vi "Grid Pattern Dialog.vi"(8 "error in (no error)":errorcluster, 10 "Fixed Shape?":bool, 11 "Grid Settings In":T1={"Grid Type"=enum."Single Point", "Complex Convention"=enum."Re / Im", "Pattern Type"=enum."Rectangular", "Major Order Index"=0, "Grid Settings Value 1"=0.0+0.0i, "Grid Settings Value 2"=0.0+0.0i, "Pattern Settings Value 1"=0, "Pattern Settings Value 2"=0, "Values"=[0.0+0.0i]}) -> (0 "error out":errorcluster, 1 "Cancelled?":bool, 2 "Values":cdb[](array[numeric]), 3 "Grid Settings Out":T1={"Grid Type"=enum."Single Point", "Complex Convention"=enum."Re / Im", "Pattern Type"=enum."Rectangular", "Major Order Index"=0, "Grid Settings Value 1"=0.0+0.0i, "Grid Settings Value 2"=0.0+0.0i, "Pattern Settings Value 1"=0, "Pattern Settings Value 2"=0, "Values"=[0.0+0.0i]})   [LabVIEW 2023, in "NI_HFNetworkAnalysis.lvlib"]
doc: "Dialog box to define a grid pattern of complex values on a Smith Chart."
uses:
  NI_HFNetworkAnalysis.lvlib
  Controls/GridSettings.ctl
  Controls/ComplexConvention.ctl
  Controls/GridPatternType.ctl
  <vilib>/Utility/miscctls.llb/LVRowAndColumnTypeDef.ctl
  <vilib>/picture/smith.llb/Smith Plot Style.ctl
panel:
  in  "Right Panel":enum32{"Page 2"}(tab)
  out "Smith Chart":picture
  in  "Left Panel":enum32{"Page 1", "Page 3"}(tab)
  in  "Grid Settings":T4 caption="Grid"
  in  "Pattern Settings":cluster{"value1":u32, "value2":u32}={"value1"=1, "value2"=1} caption="Pattern" {"value2" min=1; "value1" min=1}
  in  "Point":T5
  out "Custom Grid":string[][](table)
  in  "Cancel Button":bool
  in  "OK Button":bool
  in  "Order":u16(ring) caption="Order:" items=["Amp slowest", "Pha slowest"]
  in  "Shape Type":u16(ring) caption="Shape:" items=["Single Point", "Rectangle", "Circle", "Pie", "Custom"]
  in  "Pattern Type":u16(ring) caption="Format:" items=["Re / Im", "Amp / Pha"]
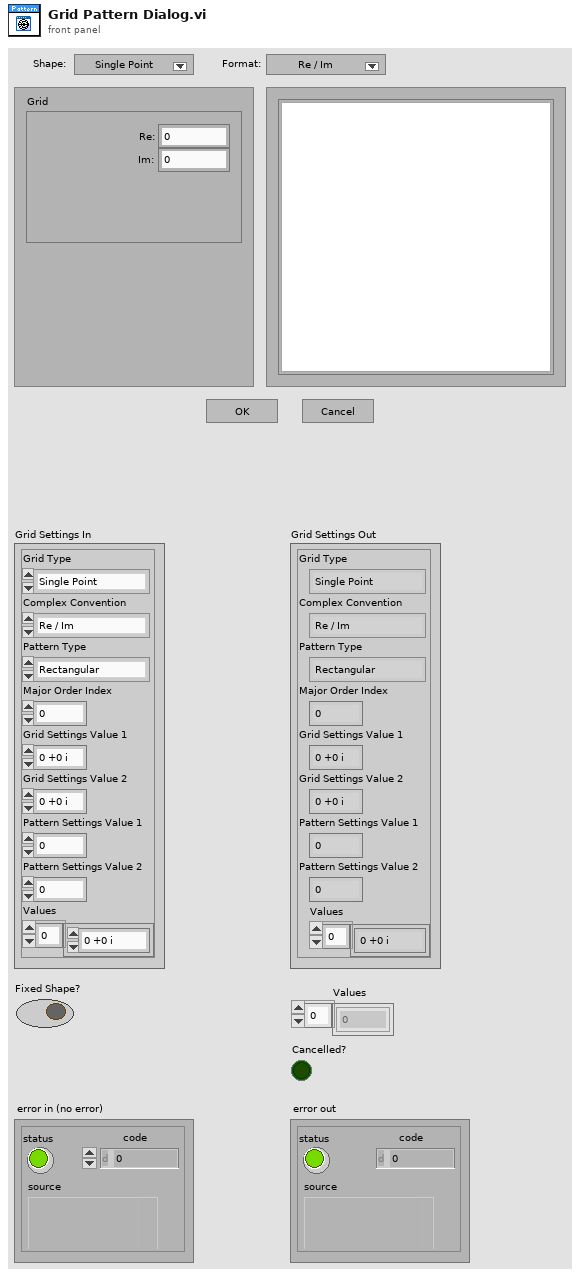
[diagram p1: front panel]
types:
  T1 = typedef "NI_HFNetworkAnalysis.lvlib/GridSettings.ctl" = cluster{"Grid Type":enum16{"Single Point", "Rectangle", "Circle", "Pie", "Custom"}, "Complex Convention":T2, "Pattern Type":T3, "Major Order Index":i32, "Grid Settings Value 1":cdb, "Grid Settings Value 2":cdb, "Pattern Settings Value 1":u32, "Pattern Settings Value 2":u32, "Values":cdb[]}
  T2 = typedef "NI_HFNetworkAnalysis.lvlib/ComplexConvention.ctl" = enum16{"Re / Im", "Amp / Pha"}
  T3 = typedef "NI_HFNetworkAnalysis.lvlib/GridPatternType.ctl" = enum16{"Rectangular", "Circular", "Undefined"}
  T4 = cluster{"value1":dbl, "value2":dbl, "value3":dbl, "value4":dbl}
  T5 = cluster{"value1":dbl, "value2":dbl, "Delete Point":bool, "Add Point":bool}
  T6 = enum16{"Single Point", "Rectangle", "Circle", "Pie", "Custom"}
  T7 = cluster{"# Horiz Points:":dbl, "# Vert Points:":dbl, "Delete Point":bool, "Add Point":bool}
  T8 = typedef "LVRowAndColumnTypeDef.ctl" = cluster{"Row":i32, "Column":i32}
  T9 = enum8{"Enabled", "Disabled", "Disabled and Grayed Out"}
  T10 = cluster{"x minimum":dbl, "x maximum":dbl, "y minimum":dbl, "y maximum":dbl}
  T11 = typedef "Smith Plot Style.ctl" = u16
  T12 = cluster{"Plot Style":T11, "Line Color":u32, "Point Color":u32}
  T13 = cluster{"R color":u32, "R grids":bool, "X color":u32, "X grids":bool, "Labels":bool}
  T14 = typedef "LVBoundsTypeDef.ctl" = cluster{"Width":u32, "Height":u32}
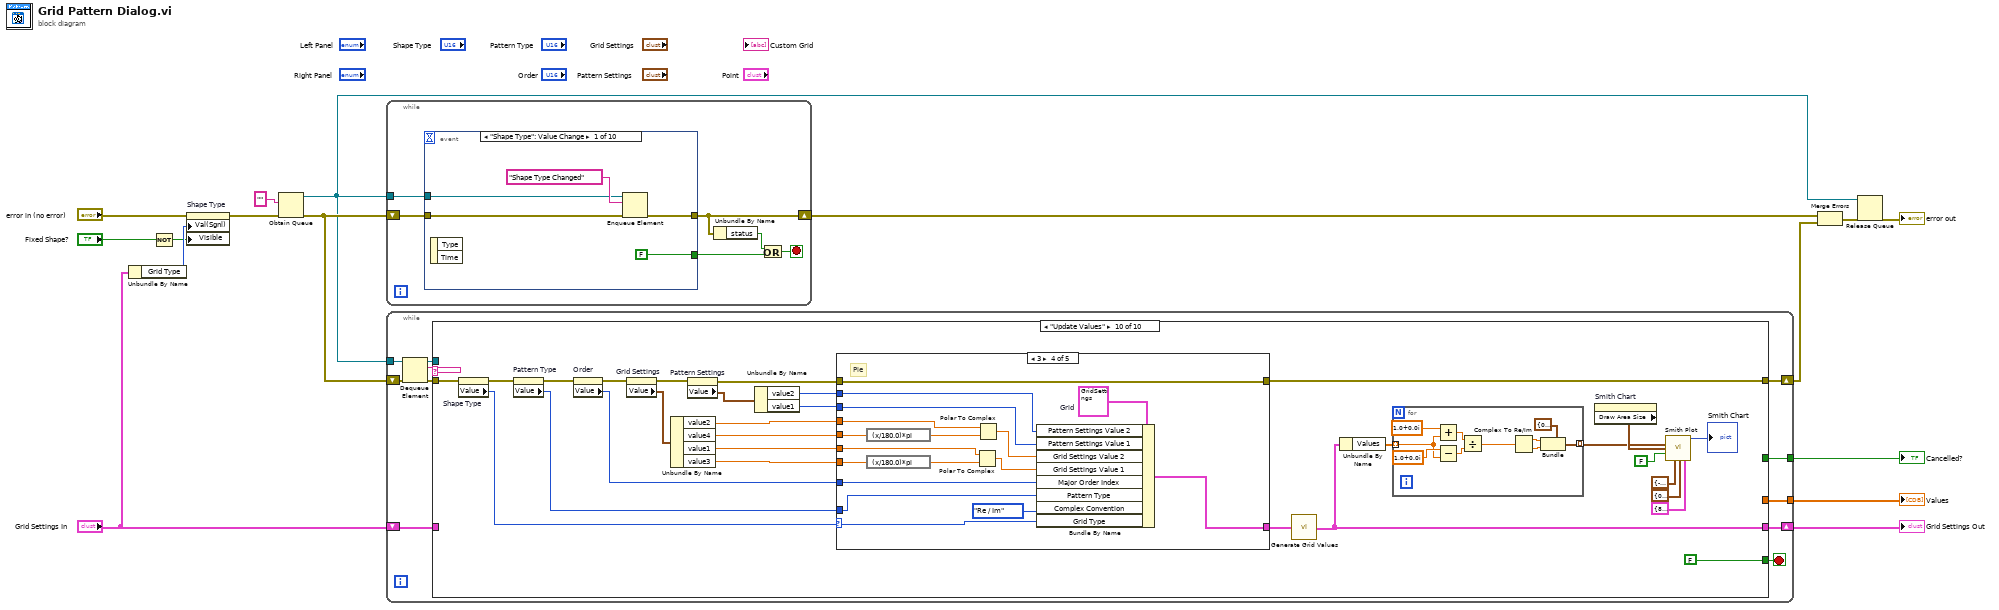
[diagram p0: block diagram]
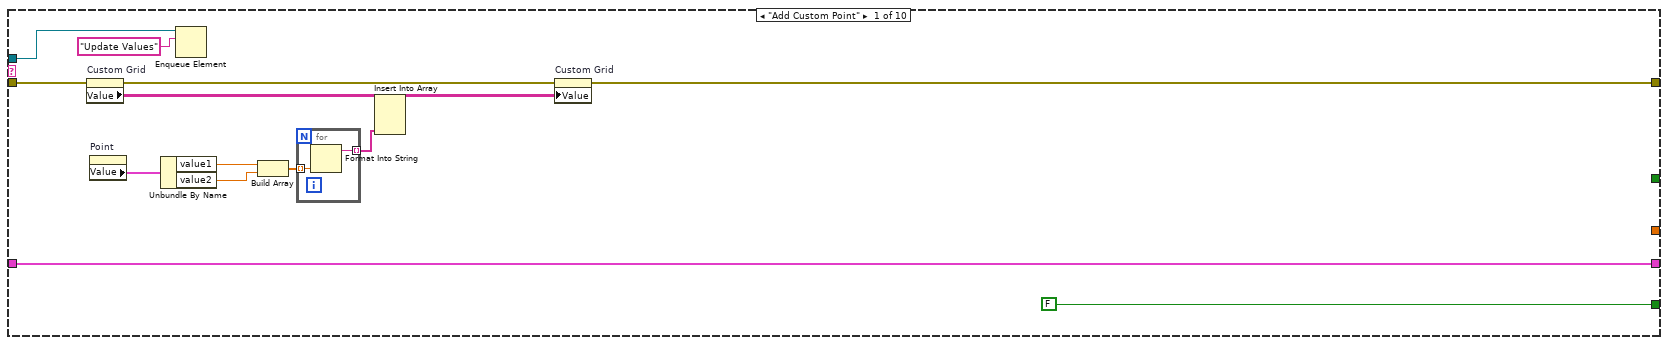
[diagram p2: hidden frame]
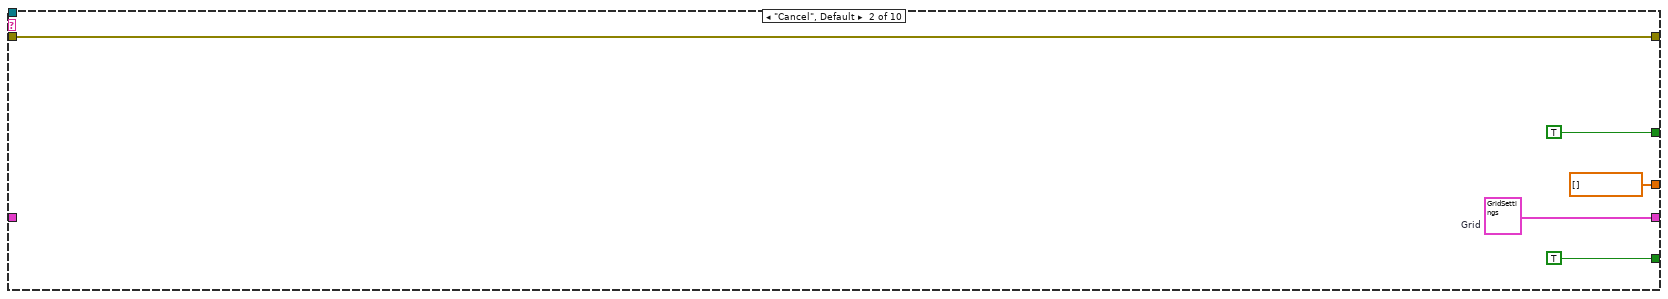
[diagram p3: hidden frame]
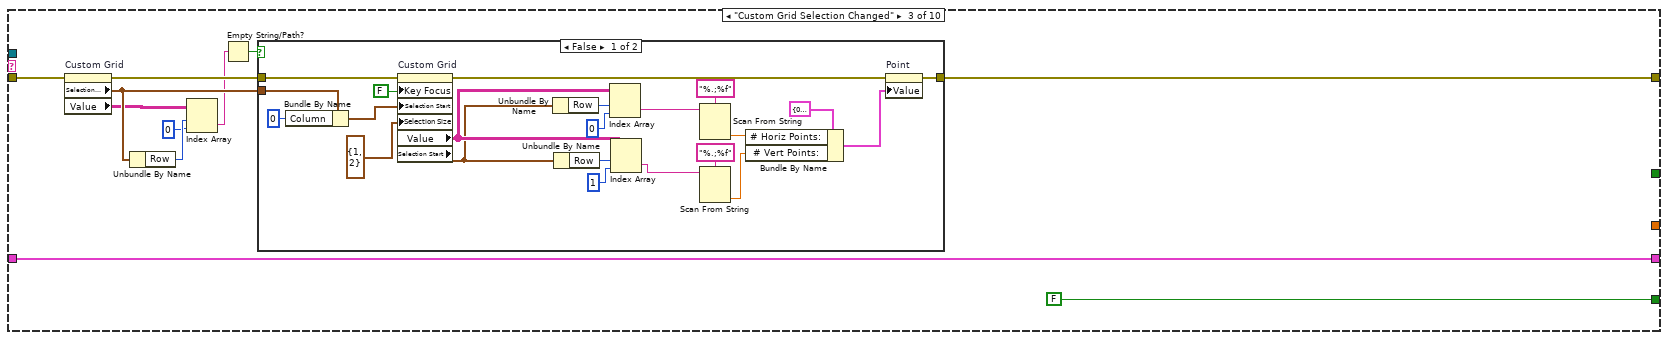
[diagram p4: hidden frame]
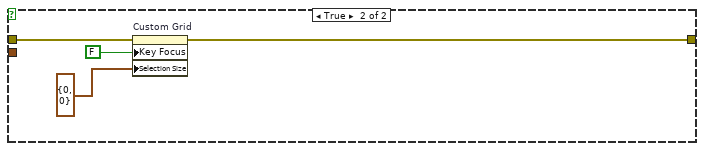
[diagram p5: hidden frame]
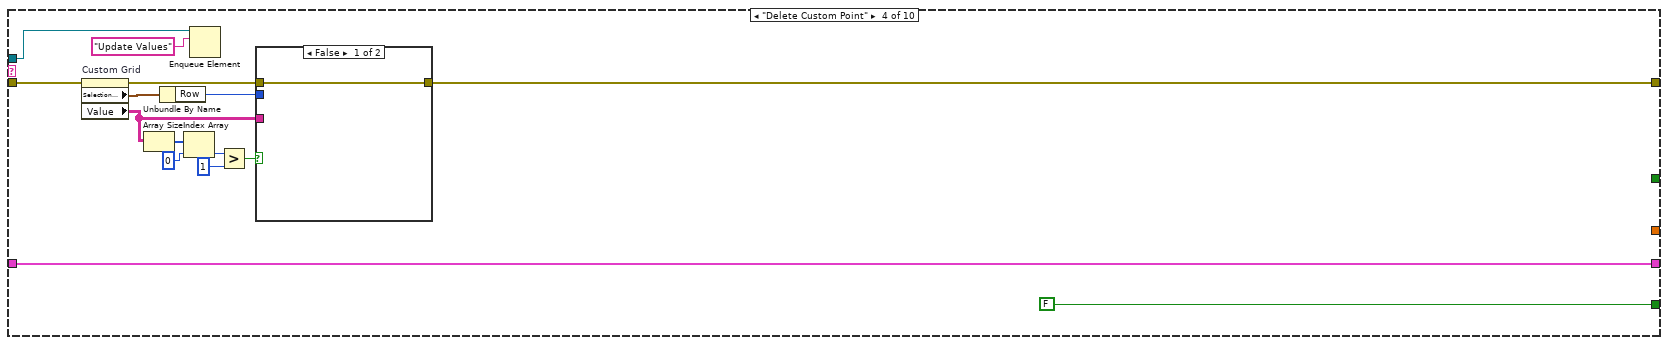
[diagram p6: hidden frame]
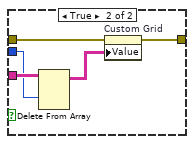
[diagram p7: hidden frame]
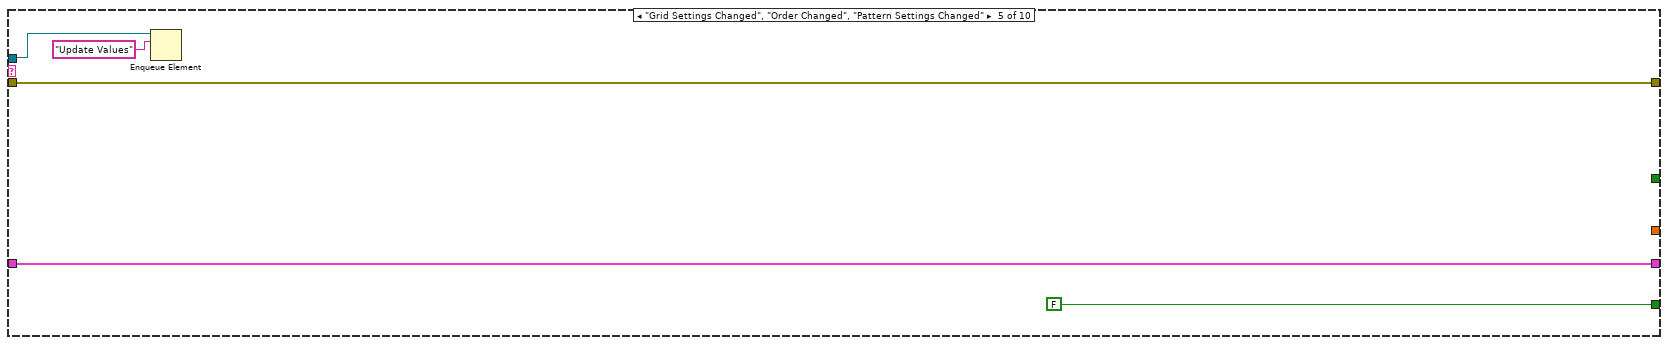
[diagram p8: hidden frame]
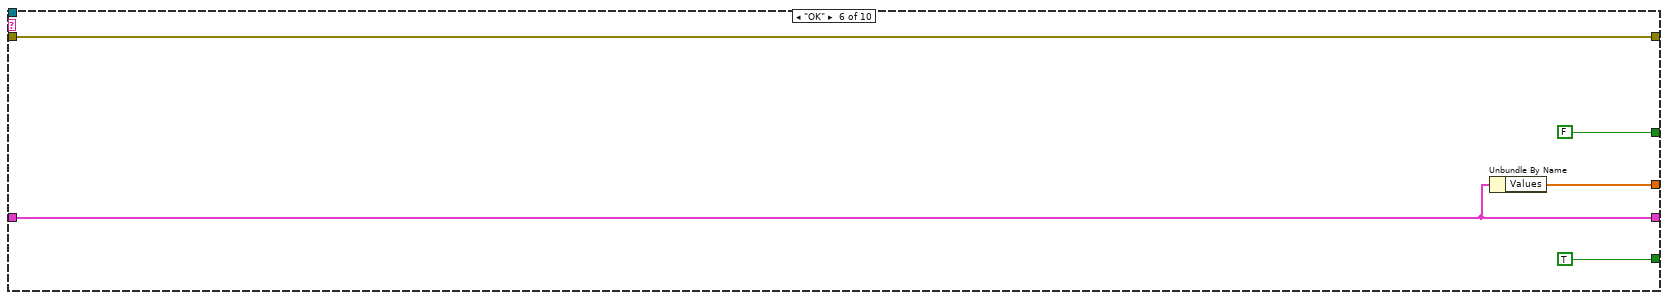
[diagram p9: hidden frame]
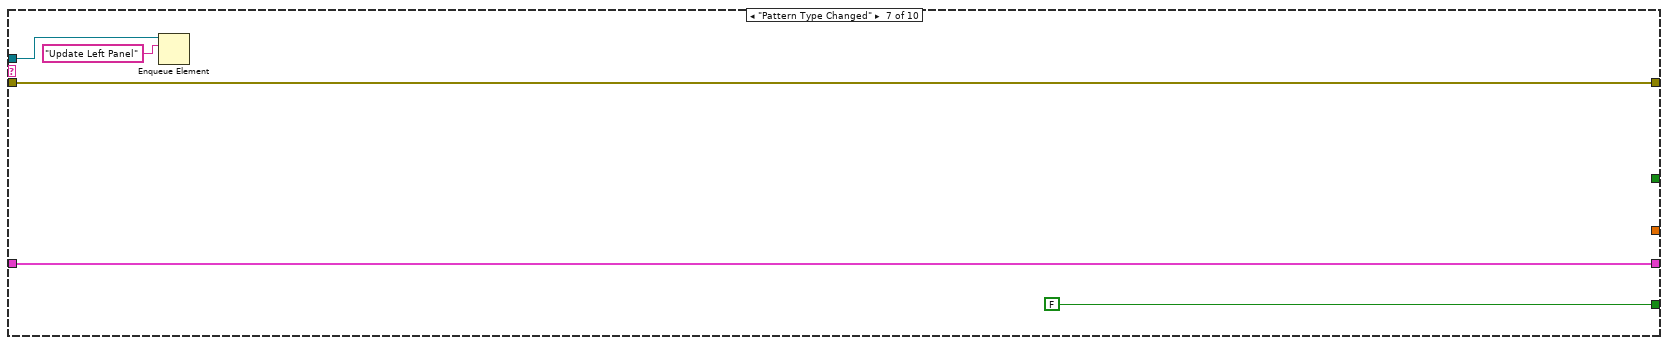
[diagram p10: hidden frame]
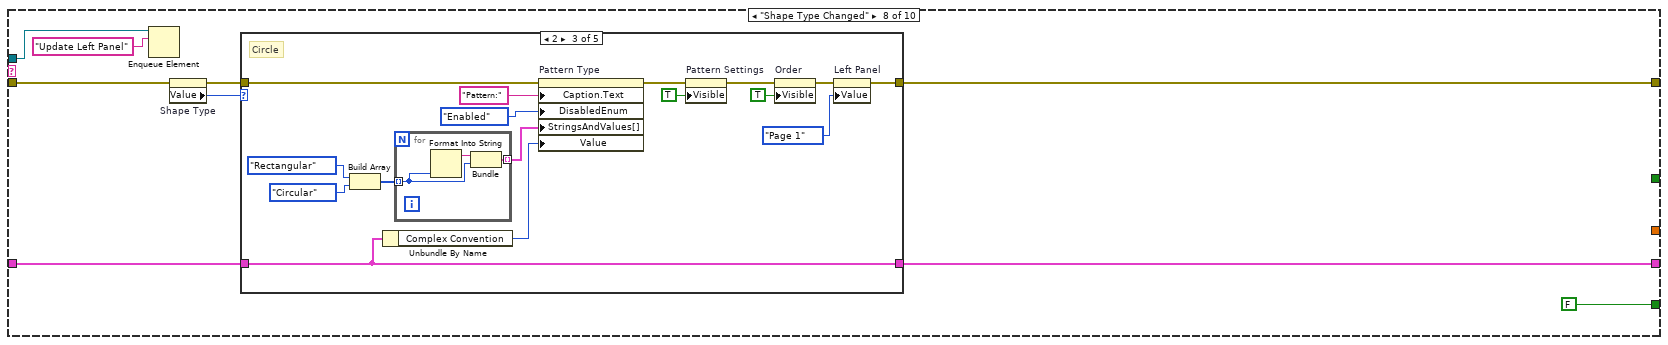
[diagram p11: hidden frame]
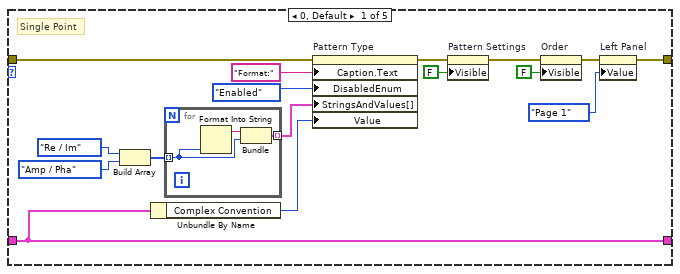
[diagram p12: hidden frame]
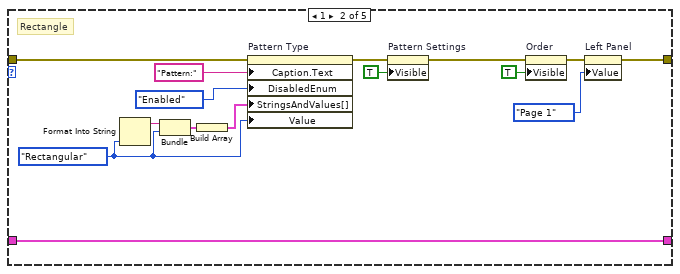
[diagram p13: hidden frame]
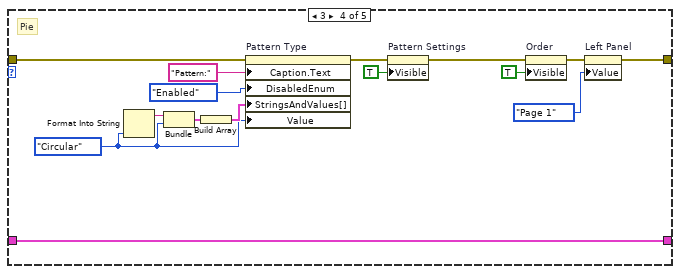
[diagram p14: hidden frame]
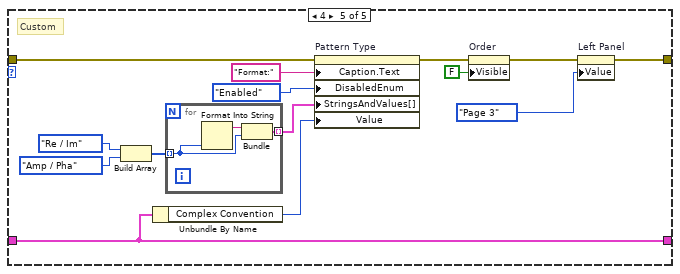
[diagram p15: hidden frame]
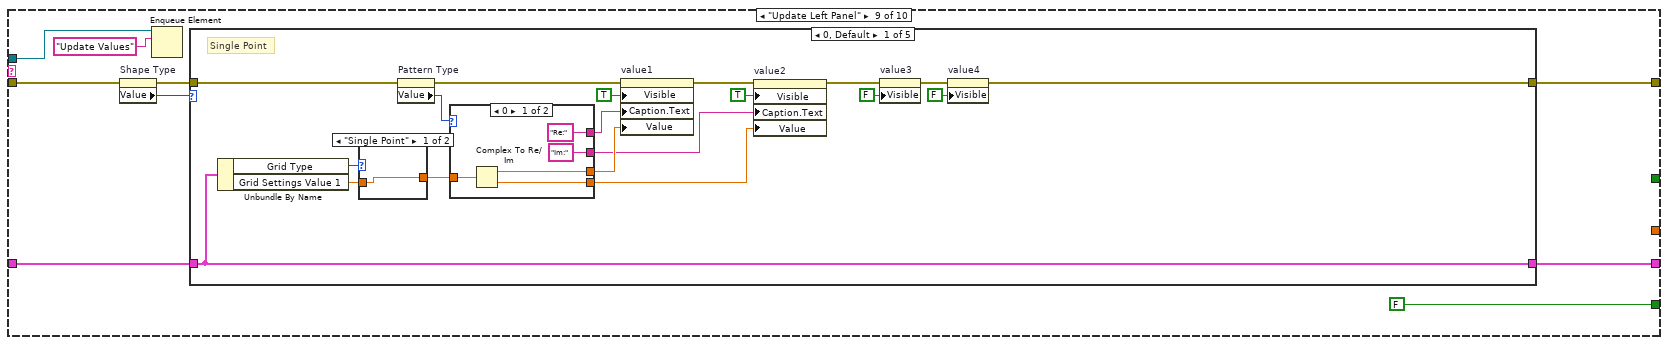
[diagram p16: hidden frame]
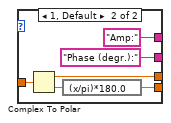
[diagram p17: hidden frame]
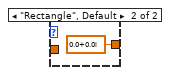
[diagram p18: hidden frame]
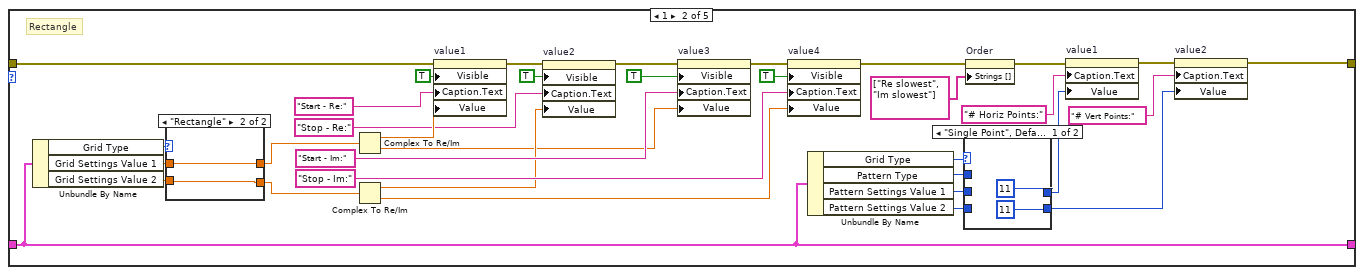
[diagram p19: hidden frame]
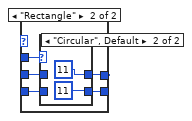
[diagram p20: hidden frame]
diagram:
  n1 = Unbundle By Name("Grid Settings In") -> ("Grid Type"=w3:T6)
  n2 = Not(x="Fixed Shape?") -> (.not. x?=w1:bool)
  n3 = property on="Shape Type" class="Ring (strict)"(error in="error in (no error)", "Val(Sgnl)"=w3, "Visible"=w1) -> (error out=w8:errorcluster)  [unwired: 1 in, 1 out]
  n4 = Obtain Queue(element data type="", error in (no error)=w8) -> (queue out=w11:refnum<queue>, error out=w15:errorcluster)  [unwired: 3 in, 1 out]
  n5 = while {
    shift-right: [w17] -> w14
    shift-left: w15 -> [w19]
    tunnel: w11 -> [w18]
    stop <- w22 stop-if-true
    n6 = event shown="[0] \"Shape Type\": Value Change" {
      selector: _ -> [_ _ _ _ _ _ _ _ _ _]
      dyn-events: _ -> [_ _ _ _ _ _ _ _ _ _]
      timeout: _ -> [_ _ _ _ _ _ _ _ _ _]
      tunnel: [FALSE FALSE FALSE FALSE FALSE FALSE FALSE FALSE TRUE TRUE] -> w20
      tunnel: w19 -> [w25 w30 w35 w40 w45 w48 w56 w66 w71 w76]
      tunnel: w18 -> [w23 w28 w33 w38 w43 w52 w60 w64 w69 w74]
      tunnel: [w26 w31 w36 w41 w46 w54 w62 w67 w72 w77] -> w17
      event "Shape Type": Value Change {
        n7 = event-data() -> ()  [unwired: 1 in, 2 out]
        n8 = Enqueue Element(queue=w23, element="Shape Type Changed", error in (no error)=w25) -> (error out=w26:errorcluster)  [unwired: 1 in, 2 out]
      }
      event "Pattern Settings": Value Change {
        n9 = event-data() -> ()  [unwired: 1 in, 2 out]
        n10 = Enqueue Element(queue=w28, element="Pattern Settings Changed", error in (no error)=w30) -> (error out=w31:errorcluster)  [unwired: 1 in, 2 out]
      }
      event "Order": Value Change {
        n11 = event-data() -> ()  [unwired: 1 in, 3 out]
        n12 = Enqueue Element(queue=w33, element="Order Changed", error in (no error)=w35) -> (error out=w36:errorcluster)  [unwired: 1 in, 2 out]
      }
      event "Custom Grid": Mouse Up {
        n13 = event-data() -> ()  [unwired: 1 in, 2 out]
        n14 = Enqueue Element(queue=w38, element="Custom Grid Selection Changed", error in (no error)=w40) -> (error out=w41:errorcluster)  [unwired: 1 in, 2 out]
      }
      event "Grid Settings": Value Change {
        n15 = event-data() -> ()  [unwired: 1 in, 2 out]
        n16 = Enqueue Element(queue=w43, element="Grid Settings Changed", error in (no error)=w45) -> (error out=w46:errorcluster)  [unwired: 1 in, 2 out]
      }
      event "Point.Add Point": Value Change {
        # "Reset Button"
        n17 = event-data() -> ("CtlRef"=w51:refnum<vi>, "OldVal"=w50:bool)  [unwired: 1 in]
        n18 = property class="Bool (strict)"(reference=w51, error in=w48, "Value"=w50) -> (error out=w49:errorcluster)  [unwired: 1 out]
        n19 = Enqueue Element(queue=w52, element="Add Custom Point", error in (no error)=w49) -> (error out=w54:errorcluster)  [unwired: 1 in, 2 out]
      }
      event "Point.Delete Point": Value Change {
        # "Reset Button"
        n20 = event-data() -> ("CtlRef"=w59:refnum<vi>, "OldVal"=w58:bool)  [unwired: 1 in]
        n21 = property class="Bool (strict)"(reference=w59, error in=w56, "Value"=w58) -> (error out=w57:errorcluster)  [unwired: 1 out]
        n22 = Enqueue Element(queue=w60, element="Delete Custom Point", error in (no error)=w57) -> (error out=w62:errorcluster)  [unwired: 1 in, 2 out]
      }
      event "Pattern Type": Value Change {
        n23 = event-data() -> ()  [unwired: 1 in, 2 out]
        n24 = Enqueue Element(queue=w64, element="Pattern Type Changed", error in (no error)=w66) -> (error out=w67:errorcluster)  [unwired: 1 in, 2 out]
      }
      event "Cancel Button": Value Change {
        n25 = event-data() -> ()  [unwired: 1 in, 2 out]
        n26 = Enqueue Element(queue=w69, element="Cancel", error in (no error)=w71) -> (error out=w72:errorcluster)  [unwired: 1 in, 2 out]
      }
      event "OK Button": Value Change {
        n27 = event-data() -> ()  [unwired: 1 in, 2 out]
        n28 = Enqueue Element(queue=w74, element="OK", error in (no error)=w76) -> (error out=w77:errorcluster)  [unwired: 1 in, 2 out]
      }
    }
    n29 = Unbundle By Name(w17) -> ("status"=w21:bool)
    n30 = Or(x=w21, y=w20) -> (x .or. y?=w22:bool)
  }
  n31 = while {
    tunnel: w11 -> [w89]
    shift-right: [w85] -> w13
    shift-left: w15 -> [w88]
    tunnel: [w82] -> w10
    shift-right: [w80] -> w5
    shift-left: "Grid Settings In" -> [w81]
    tunnel: [w79] -> w6
    stop <- w83 stop-if-true
    n32 = Dequeue Element(queue=w89, error in (no error)=w88) -> (queue out=w86:refnum<queue>, element=w84:string, error out=w87:errorcluster)  [unwired: 1 in, 1 out]
    n33 = case shown="\"Update Values\"" w84 {
      tunnel: w87 -> [w103 w109 w121 w162 w173 w177 w183 w192 w284 w589]
      tunnel: w86 -> [w93 _ _ w150 w169 _ w181 w187 w285 _]
      tunnel: [w96 w109 w119 w152 w173 w177 w183 w189 w281 w584] -> w85
      tunnel: [FALSE TRUE FALSE FALSE FALSE TRUE FALSE FALSE FALSE FALSE] -> w83
      tunnel: [_ TRUE _ _ _ FALSE _ _ _ _] -> w82
      tunnel: w81 -> [w90 _ w111 w148 w171 w175 w179 w185 w279 _]
      tunnel: [w90 w106 w111 w148 w171 w175 w179 w184 w278 w562] -> w80
      tunnel: [_ cdb[] [] ("Values") _ _ _ w174 _ _ _ _] -> w79
      frame "Add Custom Point" {
        n34 = property on="Custom Grid" class="Tbl (strict)"(error in=w103) -> (error out=w95:errorcluster, "Value"=w99:string[][])  [unwired: 1 in, 1 out]
        n35 = property on="Point" class="Clust (strict)"() -> ("Value"=w102:T5)  [unwired: 2 in, 2 out]
        n36 = Unbundle By Name(w102) -> ("value1"=w101:dbl, "value2"=w100:dbl)
        n37 = Enqueue Element(queue=w93, element="Update Values") -> ()  [unwired: 2 in, 3 out]
        n38 = Build Array(w101, w100) -> (w98:dbl[])
        n39 = for {
          tunnel: w98 -> [w105] mode=indexing
          tunnel: [w104] -> w97 mode=indexing
          n40 = Format Into String(w105) -> (resulting string=w104:string)  [unwired: 3 in, 1 out]
        }
        n41 = Insert Into Array(array=w99, new element=w97) -> (w94:string[][])  [unwired: 2 in]
        n42 = property on="Custom Grid" class="Tbl (strict)"(error in=w95, "Value"=w94) -> (error out=w96:errorcluster)  [unwired: 1 in, 1 out]
      }
      frame "Cancel", Default {
        w106 = T1 {"Grid Type"=enum."Single Point", "Complex Convention"=enum."Re / Im", "Pattern Type"=enum."Rectangular", "Major Order Index"=0, "Grid Settings Value 1"=0.0+0.0i, "Grid Settings Value 2"=0.0+0.0i, "Pattern Settings Value 1"=0, "Pattern Settings Value 2"=0, "Values"=[0.0+0.0i]}  # Grid
      }
      frame "Custom Grid Selection Changed" {
        n43 = property on="Custom Grid" class="Tbl (strict)"(error in=w121) -> (error out=w120:errorcluster, "Selection Start"=w118:T8, "Value"=w117:string[][])  [unwired: 1 in, 1 out]
        n44 = Unbundle By Name(w118) -> ("Row"=w116:i32)
        n45 = Index Array(array=w117, index (row)=w116, index (col)=0 ("disabled index (col)")) -> (element=w113:string)
        n46 = Empty String/Path?(string/path=w113) -> (empty?=w114:bool)
        n47 = case shown="False" w114 {
          tunnel: w118 -> [w141 _]
          tunnel: w120 -> [w137 w147]
          tunnel: [w123 w146] -> w119
          frame False {
            n48 = Bundle By Name(cluster=w141, "Column"=0) -> (w142:T8)
            n49 = property on="Custom Grid" class="Tbl (strict)"(error in=w137, "Key Focus"=FALSE, "Selection Start"=w142, "Selection Size"=T8 {"Row"=1, "Column"=2}) -> (error out=w122:errorcluster, "Value"=w133:string[][], "Selection Start"=w132:T8)  [unwired: 1 in, 1 out]
            n50 = Unbundle By Name(w132) -> ("Row"=w135:i32)
            n51 = Unbundle By Name(w132) -> ("Row"=w138:i32)
            n52 = Index Array(array=w133, index (row)=w135, index (col)=0 ("disabled index (col)")) -> (element=w130:string)
            n53 = Index Array(array=w133, index (row)=w138, index (col)=1 ("disabled index (col)")) -> (element=w127:string)
            n54 = Scan From String(format string="%.;%f", input string=w130) -> (output 1=w125:dbl)  [unwired: 3 in, 3 out]
            n55 = Scan From String(format string="%.;%f", input string=w127) -> (output 1=w126:dbl)  [unwired: 3 in, 3 out]
            n56 = Bundle By Name(cluster=T7 {"# Horiz Points:"=0.0, "# Vert Points:"=0.0, "Delete Point"=FALSE, "Add Point"=FALSE} ("Point"), "# Horiz Points:"=w125, "# Vert Points:"=w126) -> (w124:T7)
            n57 = property on="Point" class="Clust (strict)"(error in=w122, "Value"=w124) -> (error out=w123:errorcluster)  [unwired: 1 in, 1 out]
          }
          frame True {
            n58 = property on="Custom Grid" class="Tbl (strict)"(error in=w147, "Key Focus"=FALSE, "Selection Size"=T8 {"Row"=0, "Column"=0} ("Selection Start")) -> (error out=w146:errorcluster)  [unwired: 1 in, 1 out]
          }
        }
      }
      frame "Delete Custom Point" {
        n59 = property on="Custom Grid" class="Tbl (strict)"(error in=w162) -> (error out=w153:errorcluster, "Selection Start"=w155:T8, "Value"=w156:string[][])  [unwired: 1 in, 1 out]
        n60 = Array Size(array=w156) -> (size(s)=w161:i32[])
        n61 = Unbundle By Name(w155) -> ("Row"=w154:i32)
        n62 = Index Array(array=w161, index=0) -> (element=w159:i32)
        n63 = Enqueue Element(queue=w150, element="Update Values") -> ()  [unwired: 2 in, 3 out]
        n64 = Greater?(x=w159, y=1) -> (0:w157:bool)
        n65 = case shown="False" w157 {
          tunnel: w156 -> [_ w168]
          tunnel: w154 -> [_ w167]
          tunnel: w153 -> [w163 w166]
          tunnel: [w163 w165] -> w152
          frame False {
          }
          frame True {
            n66 = Delete From Array(array=w168, index (row)=w167) -> (array with subset deleted=w164:string[][])  [unwired: 2 in, 1 out]
            n67 = property on="Custom Grid" class="Tbl (strict)"(error in=w166, "Value"=w164) -> (error out=w165:errorcluster)  [unwired: 1 in, 1 out]
          }
        }
      }
      frame "Grid Settings Changed", "Order Changed", "Pattern Settings Changed" {
        n68 = Enqueue Element(queue=w169, element="Update Values") -> ()  [unwired: 2 in, 3 out]
      }
      frame "OK" {
        n69 = Unbundle By Name(w175) -> ("Values"=w174:cdb[])
      }
      frame "Pattern Type Changed" {
        n70 = Enqueue Element(queue=w181, element="Update Left Panel") -> ()  [unwired: 2 in, 3 out]
      }
      frame "Shape Type Changed" {
        n71 = Enqueue Element(queue=w187, element="Update Left Panel") -> ()  [unwired: 2 in, 3 out]
        n72 = property on="Shape Type" class="Ring (strict)"(error in=w192) -> (error out=w190:errorcluster, "Value"=w191:u16)  [unwired: 1 in, 1 out]
        n73 = case shown="2" w191 {
          tunnel: w190 -> [w208 w226 w233 w251 w267]
          tunnel: [w198 w217 w234 w252 w268] -> w189
          tunnel: w185 -> [w197 w216 w231 w250 w265]
          tunnel: [w197 w216 w231 w250 w265] -> w184
          frame 0, Default {
            # "Single Point"
            n74 = Build Array(ComplexConvention."Re / Im" ("ComplexConvention"), ComplexConvention."Amp / Pha" ("ComplexConvention")) -> (w196:T2[])
            n75 = Unbundle By Name(w197) -> ("Complex Convention"=w199:T2)
            n76 = for {
              tunnel: w196 -> [w210] mode=indexing
              tunnel: [w209] -> w193 mode=indexing
              n77 = Format Into String(w210) -> (resulting string=w211:string)  [unwired: 3 in, 1 out]
              n78 = Bundle(w211, "ComplexConvention"=w210) -> (w209:cluster{string, "ComplexConvention":T2})  [unwired: 1 in]
            }
            n79 = property on="Pattern Type" class="Ring (strict)"(error in=w208, "Caption.Text"="Format:" ("Label.Text"), "DisabledEnum"=T9."Enabled" ("Disabled"), "StringsAndValues[]"=w193, "Value"=w199) -> (error out=w204:errorcluster)  [unwired: 1 in, 1 out]
            n80 = property on="Pattern Settings" class="Clust (strict)"(error in=w204, "Visible"=FALSE) -> (error out=w201:errorcluster)  [unwired: 1 in, 1 out]
            n81 = property on="Order" class="Ring (strict)"(error in=w201, "Visible"=FALSE) -> (error out=w200:errorcluster)  [unwired: 1 in, 1 out]
            n82 = property on="Left Panel" class="TabCtl (strict)"(error in=w200, "Value"=enum32{"Page 1", "Page 3"}."Page 1" ("LeftPanel")) -> (error out=w198:errorcluster)  [unwired: 1 in, 1 out]
          }
          frame 1 {
            w212 = GridPatternType."Rectangular" ("GridPatternType")
            # "Rectangle"
            n83 = Format Into String(w212) -> (resulting string=w215:string)  [unwired: 3 in, 1 out]
            n84 = Bundle(w215, "GridPatternType"=w212) -> (w214:cluster{string, "GridPatternType":T3})  [unwired: 1 in]
            n85 = Build Array(w214) -> (w213:cluster{string, "GridPatternType":T3}[])
            n86 = property on="Pattern Type" class="Ring (strict)"(error in=w226, "Caption.Text"="Pattern:" ("Label.Text"), "DisabledEnum"=T9."Enabled" ("Disabled"), "StringsAndValues[]"=w213, "Value"=w212) -> (error out=w222:errorcluster)  [unwired: 1 in, 1 out]
            n87 = property on="Pattern Settings" class="Clust (strict)"(error in=w222, "Visible"=TRUE) -> (error out=w219:errorcluster)  [unwired: 1 in, 1 out]
            n88 = property on="Order" class="Ring (strict)"(error in=w219, "Visible"=TRUE) -> (error out=w218:errorcluster)  [unwired: 1 in, 1 out]
            n89 = property on="Left Panel" class="TabCtl (strict)"(error in=w218, "Value"=enum32{"Page 1", "Page 3"}."Page 1" ("LeftPanel")) -> (error out=w217:errorcluster)  [unwired: 1 in, 1 out]
          }
          frame 2 {
            # "Circle"
            n90 = Build Array(GridPatternType."Rectangular" ("GridPatternType"), GridPatternType."Circular" ("GridPatternType")) -> (w230:T3[])
            n91 = Unbundle By Name(w231) -> ("Complex Convention"=w232:T2)
            n92 = for {
              tunnel: w230 -> [w244] mode=indexing
              tunnel: [w243] -> w229 mode=indexing
              n93 = Format Into String(w244) -> (resulting string=w245:string)  [unwired: 3 in, 1 out]
              n94 = Bundle(w245, "GridPatternType"=w244) -> (w243:cluster{string, "GridPatternType":T3})  [unwired: 1 in]
            }
            n95 = property on="Pattern Type" class="Ring (strict)"(error in=w233, "Caption.Text"="Pattern:" ("Label.Text"), "DisabledEnum"=T9."Enabled" ("Disabled"), "StringsAndValues[]"=w229, "Value"=w232) -> (error out=w239:errorcluster)  [unwired: 1 in, 1 out]
            n96 = property on="Pattern Settings" class="Clust (strict)"(error in=w239, "Visible"=TRUE) -> (error out=w236:errorcluster)  [unwired: 1 in, 1 out]
            n97 = property on="Order" class="Ring (strict)"(error in=w236, "Visible"=TRUE) -> (error out=w235:errorcluster)  [unwired: 1 in, 1 out]
            n98 = property on="Left Panel" class="TabCtl (strict)"(error in=w235, "Value"=enum32{"Page 1", "Page 3"}."Page 1" ("LeftPanel")) -> (error out=w234:errorcluster)  [unwired: 1 in, 1 out]
          }
          frame 3 {
            w246 = GridPatternType."Circular" ("GridPatternType")
            # "Pie"
            n99 = Format Into String(w246) -> (resulting string=w249:string)  [unwired: 3 in, 1 out]
            n100 = Bundle(w249, "GridPatternType"=w246) -> (w248:cluster{string, "GridPatternType":T3})  [unwired: 1 in]
            n101 = Build Array(w248) -> (w247:cluster{string, "GridPatternType":T3}[])
            n102 = property on="Pattern Type" class="Ring (strict)"(error in=w251, "Caption.Text"="Pattern:" ("Label.Text"), "DisabledEnum"=T9."Enabled" ("Disabled"), "StringsAndValues[]"=w247, "Value"=w246) -> (error out=w257:errorcluster)  [unwired: 1 in, 1 out]
            n103 = property on="Pattern Settings" class="Clust (strict)"(error in=w257, "Visible"=TRUE) -> (error out=w254:errorcluster)  [unwired: 1 in, 1 out]
            n104 = property on="Order" class="Ring (strict)"(error in=w254, "Visible"=TRUE) -> (error out=w253:errorcluster)  [unwired: 1 in, 1 out]
            n105 = property on="Left Panel" class="TabCtl (strict)"(error in=w253, "Value"=enum32{"Page 1", "Page 3"}."Page 1" ("LeftPanel")) -> (error out=w252:errorcluster)  [unwired: 1 in, 1 out]
          }
          frame 4 {
            # "Custom"
            n106 = Build Array(ComplexConvention."Re / Im" ("ComplexConvention"), ComplexConvention."Amp / Pha" ("ComplexConvention")) -> (w264:T2[])
            n107 = Unbundle By Name(w265) -> ("Complex Convention"=w266:T2)
            n108 = for {
              tunnel: w264 -> [w276] mode=indexing
              tunnel: [w275] -> w261 mode=indexing
              n109 = Format Into String(w276) -> (resulting string=w277:string)  [unwired: 3 in, 1 out]
              n110 = Bundle(w277, "ComplexConvention"=w276) -> (w275:cluster{string, "ComplexConvention":T2})  [unwired: 1 in]
            }
            n111 = property on="Pattern Type" class="Ring (strict)"(error in=w267, "Caption.Text"="Format:" ("Label.Text"), "DisabledEnum"=T9."Enabled" ("Disabled"), "StringsAndValues[]"=w261, "Value"=w266) -> (error out=w271:errorcluster)  [unwired: 1 in, 1 out]
            n112 = property on="Order" class="Ring (strict)"(error in=w271, "Visible"=FALSE) -> (error out=w269:errorcluster)  [unwired: 1 in, 1 out]
            n113 = property on="Left Panel" class="TabCtl (strict)"(error in=w269, "Value"=enum32{"Page 1", "Page 3"}."Page 3" ("LeftPanel")) -> (error out=w268:errorcluster)  [unwired: 1 in, 1 out]
          }
        }
      }
      frame "Update Left Panel" {
        n114 = property on="Shape Type" class="Ring (strict)"(error in=w284) -> (error out=w282:errorcluster, "Value"=w283:u16)  [unwired: 1 in, 1 out]
        n115 = Enqueue Element(queue=w285, element="Update Values") -> ()  [unwired: 2 in, 3 out]
        n116 = case shown="0, Default" w283 {
          tunnel: w282 -> [w296 w344 w381 w489 w532]
          tunnel: [w290 w323 w374 w464 w523] -> w281
          tunnel: w279 -> [w288 w320 w370 w462 w517]
          tunnel: [w288 w320 w370 w462 w517] -> w278
          frame 0, Default {
            # "Single Point"
            n117 = Unbundle By Name(w288) -> ("Grid Type"=w287:T6, "Grid Settings Value 1"=w298:cdb)
            n118 = case shown="\"Single Point\"" w287 {
              tunnel: [w317 cdb 0.0+0.0i] -> w297
              tunnel: w298 -> [w317 _]
              frame "Single Point" {
              }
              frame "Rectangle", Default {
              }
            }
            n119 = property on="Pattern Type" class="Ring (strict)"(error in=w296) -> (error out=w289:errorcluster, "Value"=w295:u16)  [unwired: 1 in, 1 out]
            n120 = case shown="0" w295 {
              tunnel: w297 -> [w310 w314]
              tunnel: [w309 w313] -> w293
              tunnel: [w308 w311] -> w291
              tunnel: ["Re:" "Amp:"] -> w294
              tunnel: ["Im:" "Phase (degr.):"] -> w292
              frame 0 {
                n121 = Complex To Re/Im(x + iy=w310) -> (x=w309:dbl, y=w308:dbl)
              }
              frame 1, Default {
                n122 = Complex To Polar(r * e^(i*theta)=w314) -> (r=w313:dbl, theta=w312:dbl)
                n123 = expression code="(x/pi)*180.0" ("radians to degrees")(w312) -> (w311:dbl)
              }
            }
            n124 = property on="value1" class="DigNum (strict)"(error in=w289, "Visible"=TRUE, "Caption.Text"=w294, "Value"=w293) -> (error out=w303:errorcluster)  [unwired: 1 in, 1 out]
            n125 = property on="value2" class="DigNum (strict)"(error in=w303, "Visible"=TRUE, "Caption.Text"=w292, "Value"=w291) -> (error out=w299:errorcluster)  [unwired: 1 in, 1 out]
            n126 = property on="value3" class="DigNum (strict)"(error in=w299, "Visible"=FALSE) -> (error out=w300:errorcluster)  [unwired: 1 in, 1 out]
            n127 = property on="value4" class="DigNum (strict)"(error in=w300, "Visible"=FALSE) -> (error out=w290:errorcluster)  [unwired: 1 in, 1 out]
          }
          frame 1 {
            # "Rectangle"
            n128 = Unbundle By Name(w320) -> ("Grid Type"=w319:T6, "Grid Settings Value 1"=w346:cdb, "Grid Settings Value 2"=w340:cdb)
            n129 = case shown="\"Rectangle\"" w319 {
              tunnel: [cdb -0.5+0.5i ("gridSettingsValue 1") w368] -> w345
              tunnel: w346 -> [_ w368]
              tunnel: w340 -> [_ w367]
              tunnel: [cdb 0.5-0.5i ("gridSettingsValue 2") w367] -> w339
              frame "Single Point", Default {
              }
              frame "Rectangle" {
              }
            }
            n130 = Complex To Re/Im(x + iy=w345) -> (x=w342:dbl, y=w335:dbl)
            n131 = Complex To Re/Im(x + iy=w339) -> (x=w336:dbl, y=w334:dbl)
            n132 = property on="value1" class="DigNum (strict)"(error in=w344, "Visible"=TRUE, "Caption.Text"="Start - Re:", "Value"=w342) -> (error out=w351:errorcluster)  [unwired: 1 in, 1 out]
            n133 = property on="value2" class="DigNum (strict)"(error in=w351, "Visible"=TRUE, "Caption.Text"="Stop - Re:", "Value"=w336) -> (error out=w347:errorcluster)  [unwired: 1 in, 1 out]
            n134 = property on="value3" class="DigNum (strict)"(error in=w347, "Visible"=TRUE, "Caption.Text"="Start - Im:", "Value"=w335) -> (error out=w348:errorcluster)  [unwired: 1 in, 1 out]
            n135 = property on="value4" class="DigNum (strict)"(error in=w348, "Visible"=TRUE, "Caption.Text"="Stop - Im:", "Value"=w334) -> (error out=w328:errorcluster)  [unwired: 1 in, 1 out]
            n136 = Unbundle By Name(w320) -> ("Grid Type"=w330:T6, "Pattern Type"=w333:T3, "Pattern Settings Value 1"=w332:u32, "Pattern Settings Value 2"=w331:u32)
            n137 = case shown="\"Single Point\", Default" w330 {
              tunnel: w333 -> [_ w356]
              tunnel: w332 -> [_ w358]
              tunnel: [u32 11 ("patternSettingsValue 1") w360] -> w326
              tunnel: w331 -> [_ w357]
              tunnel: [u32 11 ("patternSettingsValue 2") w359] -> w322
              frame "Single Point", Default {
              }
              frame "Rectangle" {
                n138 = case shown="\"Circular\", Default" w356 {
                  tunnel: [w362 u32 11 ("patternSettingsValue 1")] -> w360
                  tunnel: [w361 u32 11 ("patternSettingsValue 2")] -> w359
                  tunnel: w357 -> [w361 _]
                  tunnel: w358 -> [w362 _]
                  frame "Rectangular" {
                  }
                  frame "Circular", Default {
                  }
                }
              }
            }
            n139 = property on="Order" class="Ring (strict)"(error in=w328, "Strings []"=string[] ["Re slowest", "Im slowest"]) -> (error out=w325:errorcluster)  [unwired: 1 in, 1 out]
            n140 = property on="value1" class="DigNum (strict)"(error in=w325, "Caption.Text"="# Horiz Points:", "Value"=w326) -> (error out=w324:errorcluster)  [unwired: 1 in, 1 out]
            n141 = property on="value2" class="DigNum (strict)"(error in=w324, "Caption.Text"="# Vert Points:", "Value"=w322) -> (error out=w323:errorcluster)  [unwired: 1 in, 1 out]
          }
          frame 2 {
            # "Circle"
            n142 = Unbundle By Name(w370) -> ("Grid Type"=w369:T6, "Grid Settings Value 1"=w391:cdb, "Grid Settings Value 2"=w386:cdb)
            n143 = case shown="\"Single Point\", Default" w369 {
              tunnel: [cdb 0.0+0.0i ("gridSettingsValue 1") w461] -> w390
              tunnel: w391 -> [_ w461]
              tunnel: w386 -> [_ w460]
              tunnel: [cdb 0.5+0.0i ("gridSettingsValue 2") w460] -> w384
              frame "Single Point", Default {
              }
              frame "Circle" {
              }
            }
            n144 = property on="Pattern Type" class="Ring (strict)"(error in=w381) -> (error out=w380:errorcluster, "Value"=w379:u16)  [unwired: 1 in, 1 out]
            n145 = case shown="0" w379 {
              tunnel: w390 -> [w451 w457]
              tunnel: ["Center - Re:" "Center - Amp:"] -> w389
              tunnel: [w449 w456] -> w388
              tunnel: ["Center - Im:" "Center - Pha (degr.):"] -> w387
              tunnel: [w447 w454] -> w383
              frame 0 {
                n146 = Complex To Re/Im(x + iy=w451) -> (x=w449:dbl, y=w447:dbl)
              }
              frame 1, Default {
                n147 = Complex To Polar(r * e^(i*theta)=w457) -> (r=w456:dbl, theta=w455:dbl)
                n148 = expression code="(x/pi)*180.0" ("radians to degrees")(w455) -> (w454:dbl)
              }
            }
            n149 = Absolute Value(x=w384) -> (abs(x)=w382:dbl)
            n150 = property on="value1" class="DigNum (strict)"(error in=w380, "Visible"=TRUE, "Caption.Text"=w389, "Value"=w388) -> (error out=w396:errorcluster)  [unwired: 1 in, 1 out]
            n151 = property on="value2" class="DigNum (strict)"(error in=w396, "Visible"=TRUE, "Caption.Text"=w387, "Value"=w383) -> (error out=w392:errorcluster)  [unwired: 1 in, 1 out]
            n152 = property on="value3" class="DigNum (strict)"(error in=w392, "Visible"=TRUE, "Caption.Text"="Radius:", "Value"=w382) -> (error out=w393:errorcluster)  [unwired: 1 in, 1 out]
            n153 = Unbundle By Name(w370) -> ("Grid Type"=w375:T6, "Pattern Type"=w378:T3, "Pattern Settings Value 1"=w377:u32, "Pattern Settings Value 2"=w376:u32)
            n154 = property on="value4" class="DigNum (strict)"(error in=w393, "Visible"=FALSE) -> (error out=w373:errorcluster)  [unwired: 1 in, 1 out]
            n155 = property on="Pattern Type" class="Ring (strict)"(error in=w373) -> (error out=w372:errorcluster, "Value"=w371:u16)  [unwired: 1 in, 1 out]
            n156 = case shown="1" w371 {
              tunnel: w378 -> [w411 w435]
              tunnel: w377 -> [w410 w434]
              tunnel: w376 -> [w409 w433]
              tunnel: w375 -> [w408 w432]
              tunnel: [w400 w424] -> w374
              tunnel: w372 -> [w399 w423]
              frame 0, Default {
                n157 = case shown="\"Circle\"" w408 {
                  tunnel: w411 -> [_ w414]
                  tunnel: w410 -> [_ w416]
                  tunnel: [u32 11 ("patternSettingsValue 1") w418] -> w405
                  tunnel: w409 -> [_ w415]
                  tunnel: [u32 11 ("patternSettingsValue 2") w417] -> w402
                  frame "Single Point", Default {
                  }
                  frame "Circle" {
                    n158 = case shown="\"Circular\", Default" w414 {
                      tunnel: [w420 u32 11 ("patternSettingsValue 1")] -> w418
                      tunnel: [w419 u32 11 ("patternSettingsValue 2")] -> w417
                      tunnel: w415 -> [w419 _]
                      tunnel: w416 -> [w420 _]
                      frame "Rectangular" {
                      }
                      frame "Circular", Default {
                      }
                    }
                  }
                }
                n159 = property on="Order" class="Ring (strict)"(error in=w399, "Strings []"=string[] ["Re slowest", "Im slowest"]) -> (error out=w404:errorcluster)  [unwired: 1 in, 1 out]
                n160 = property on="value1" class="DigNum (strict)"(error in=w404, "Caption.Text"="# Horiz Points:", "Value"=w405) -> (error out=w403:errorcluster)  [unwired: 1 in, 1 out]
                n161 = property on="value2" class="DigNum (strict)"(error in=w403, "Caption.Text"="# Vert Points:", "Value"=w402) -> (error out=w400:errorcluster)  [unwired: 1 in, 1 out]
              }
              frame 1 {
                n162 = case shown="\"Circle\"" w432 {
                  tunnel: w435 -> [_ w438]
                  tunnel: w434 -> [_ w440]
                  tunnel: [u32 6 ("patternSettingsValue 1") w442] -> w429
                  tunnel: w433 -> [_ w439]
                  tunnel: [u32 12 ("patternSettingsValue 2") w441] -> w426
                  frame "Single Point", Default {
                  }
                  frame "Circle" {
                    n163 = case shown="\"Circular\"" w438 {
                      tunnel: [w444 u32 6 ("patternSettingsValue 1")] -> w442
                      tunnel: [w443 u32 12 ("patternSettingsValue 2")] -> w441
                      tunnel: w439 -> [w443 _]
                      tunnel: w440 -> [w444 _]
                      frame "Circular" {
                      }
                      frame "Rectangular", Default {
                      }
                    }
                  }
                }
                n164 = property on="Order" class="Ring (strict)"(error in=w423, "Strings []"=string[] ["Amp slowest", "Pha slowest"]) -> (error out=w428:errorcluster)  [unwired: 1 in, 1 out]
                n165 = property on="value1" class="DigNum (strict)"(error in=w428, "Caption.Text"="# Circles:", "Value"=w429) -> (error out=w427:errorcluster)  [unwired: 1 in, 1 out]
                n166 = property on="value2" class="DigNum (strict)"(error in=w427, "Caption.Text"="# Angles:", "Value"=w426) -> (error out=w424:errorcluster)  [unwired: 1 in, 1 out]
              }
            }
          }
          frame 3 {
            # "Pie"
            n167 = Unbundle By Name(w462) -> ("Grid Type"=w463:T6, "Grid Settings Value 1"=w491:cdb, "Grid Settings Value 2"=w485:cdb)
            n168 = case shown="\"Single Point\", Default" w463 {
              tunnel: [cdb 0.7+0.0i ("gridSettingsValue 1") w515] -> w490
              tunnel: w491 -> [_ w515]
              tunnel: w485 -> [_ w514]
              tunnel: [w512 w514] -> w484
              frame "Single Point", Default {
                n169 = Polar To Complex(1:1.5707963267948966, 2:1.0 ("r")) -> (0:w512:cdb)
              }
              frame "Pie" {
              }
            }
            n170 = Complex To Polar(r * e^(i*theta)=w490) -> (r=w487:dbl, theta=w480:dbl)
            n171 = Complex To Polar(r * e^(i*theta)=w484) -> (r=w481:dbl, theta=w478:dbl)
            n172 = property on="value1" class="DigNum (strict)"(error in=w489, "Visible"=TRUE, "Caption.Text"="Radius - Min:", "Value"=w487) -> (error out=w496:errorcluster)  [unwired: 1 in, 1 out]
            n173 = expression code="(x/pi)*180.0" ("radians to degrees")(w480) -> (w479:dbl)
            n174 = property on="value2" class="DigNum (strict)"(error in=w496, "Visible"=TRUE, "Caption.Text"="Radius - Max:", "Value"=w481) -> (error out=w492:errorcluster)  [unwired: 1 in, 1 out]
            n175 = expression code="(x/pi)*180.0" ("radians to degrees")(w478) -> (w477:dbl)
            n176 = property on="value3" class="DigNum (strict)"(error in=w492, "Visible"=TRUE, "Caption.Text"="Angle (degr.) - Start:", "Value"=w479) -> (error out=w493:errorcluster)  [unwired: 1 in, 1 out]
            n177 = property on="value4" class="DigNum (strict)"(error in=w493, "Visible"=TRUE, "Caption.Text"="Angle (degr.) - Stop:", "Value"=w477) -> (error out=w469:errorcluster)  [unwired: 1 in, 1 out]
            n178 = Unbundle By Name(w462) -> ("Grid Type"=w468:T6, "Pattern Type"=w467:T3, "Pattern Settings Value 1"=w466:u32, "Pattern Settings Value 2"=w465:u32)
            n179 = case shown="\"Pie\"" w468 {
              tunnel: w467 -> [_ w501]
              tunnel: w466 -> [_ w503]
              tunnel: [u32 6 ("patternSettingsValue 1") w505] -> w474
              tunnel: w465 -> [_ w502]
              tunnel: [u32 12 ("patternSettingsValue 2") w504] -> w471
              frame "Single Point", Default {
              }
              frame "Pie" {
                n180 = case shown="\"Rectangular\", Default" w501 {
                  tunnel: [w507 u32 6 ("patternSettingsValue 1")] -> w505
                  tunnel: [w506 u32 12 ("patternSettingsValue 2")] -> w504
                  tunnel: w502 -> [w506 _]
                  tunnel: w503 -> [w507 _]
                  frame "Circular" {
                  }
                  frame "Rectangular", Default {
                  }
                }
              }
            }
            n181 = property on="Order" class="Ring (strict)"(error in=w469, "Strings []"=string[] ["Amp slowest", "Pha slowest"]) -> (error out=w473:errorcluster)  [unwired: 1 in, 1 out]
            n182 = property on="value1" class="DigNum (strict)"(error in=w473, "Caption.Text"="# Circles:", "Value"=w474) -> (error out=w472:errorcluster)  [unwired: 1 in, 1 out]
            n183 = property on="value2" class="DigNum (strict)"(error in=w472, "Caption.Text"="# Angles:", "Value"=w471) -> (error out=w464:errorcluster)  [unwired: 1 in, 1 out]
          }
          frame 4 {
            # "Custom"
            n184 = Unbundle By Name(w517) -> ("Values"=w516:cdb[])
            n185 = Empty Array?(array=w516) -> (empty?=w533:bool)
            n186 = case shown="False" w533 {
              tunnel: [cdb[] [0.0+0.0i] w560] -> w530
              tunnel: w516 -> [_ w560]
              frame True {
              }
              frame False {
              }
            }
            n187 = property on="Pattern Type" class="Ring (strict)"(error in=w532) -> (error out=w528:errorcluster, "Value"=w531:u16)  [unwired: 1 in, 1 out]
            n188 = case shown="0, Default" w531 {
              tunnel: w530 -> [w535 w549]
              tunnel: ["Re" "Amp"] -> w521
              tunnel: ["Im" "Pha (degr.)"] -> w518
              tunnel: [w534 w546] -> w527
              frame 0, Default {
                n189 = for {
                  tunnel: w535 -> [w545] mode=indexing
                  tunnel: [w544] -> w534 mode=indexing
                  n190 = Complex To Re/Im(x + iy=w545) -> (x=w543:dbl, y=w538:dbl)
                  n191 = Format Into String(format string="%.;%#.5f", w543) -> (resulting string=w541:string)  [unwired: 2 in, 1 out]
                  n192 = Format Into String(format string="%.;%#.5f", w538) -> (resulting string=w539:string)  [unwired: 2 in, 1 out]
                  n193 = Build Array(w541, w539) -> (w544:string[])
                }
              }
              frame 1 {
                n194 = for {
                  tunnel: w549 -> [w558] mode=indexing
                  tunnel: [w557] -> w546 mode=indexing
                  n195 = Complex To Polar(r * e^(i*theta)=w558) -> (r=w555:dbl, theta=w556:dbl)
                  n196 = expression code="(x/pi)*180.0" ("radians to degrees")(w556) -> (w551:dbl)
                  n197 = Format Into String(format string="%#.5f", w555) -> (resulting string=w553:string)  [unwired: 2 in, 1 out]
                  n198 = Format Into String(format string="%#.1f", w551) -> (resulting string=w550:string)  [unwired: 2 in, 1 out]
                  n199 = Build Array(w553, w550) -> (w557:string[])
                }
              }
            }
            n200 = Build Array(w521, w518) -> (w529:string[])
            n201 = property on="Custom Grid" class="Tbl (strict)"(error in=w528, "Column Headers[]"=w529, "Value"=w527) -> (error out=w525:errorcluster)  [unwired: 1 in, 1 out]
            n202 = Concatenate Strings(w521, ":" ("string")) -> (w526:string)
            n203 = property on="value1" class="DigNum (strict)"(error in=w525, "Caption.Text"=w526) -> (error out=w524:errorcluster)  [unwired: 1 in, 1 out]
            n204 = Concatenate Strings(w518, ":" ("string")) -> (w519:string)
            n205 = property on="value2" class="DigNum (strict)"(error in=w524, "Caption.Text"=w519) -> (error out=w523:errorcluster)  [unwired: 1 in, 1 out]
          }
        }
      }
      frame "Update Values" {
        n206 = property on="Shape Type" class="Ring (strict)"(error in=w589) -> (error out=w582:errorcluster, "Value"=w571:u16)  [unwired: 1 in, 1 out]
        n207 = property on="Pattern Type" class="Ring (strict)"(error in=w582) -> (error out=w580:errorcluster, "Value"=w578:u16)  [unwired: 1 in, 1 out]
        n208 = property on="Order" class="Ring (strict)"(error in=w580) -> (error out=w579:errorcluster, "Value"=w577:u16)  [unwired: 1 in, 1 out]
        n209 = property on="Grid Settings" class="Clust (strict)"(error in=w579) -> (error out=w581:errorcluster, "Value"=w576:T4)  [unwired: 1 in, 1 out]
        n210 = Unbundle By Name(w576) -> ("value2"=w567:dbl, "value4"=w568:dbl, "value1"=w569:dbl, "value3"=w570:dbl)
        n211 = property on="Pattern Settings" class="Clust (strict)"(error in=w581) -> (error out=w572:errorcluster, "Value"=w575:cluster{"value1":u32, "value2":u32})  [unwired: 1 in, 1 out]
        n212 = Unbundle By Name(w575) -> ("value2"=w574:u32, "value1"=w573:u32)
        n213 = case shown="3" w571 {
          selector: w571 -> [w608 w631 w643 w667 w675]
          tunnel: w572 -> [w612 w634 w646 w670 w677]
          tunnel: [w612 w634 w646 w670 w676] -> w584
          tunnel: [w601 w633 w645 w669 w674] -> w563
          tunnel: w578 -> [w607 w621 w641 w661 w673]
          tunnel: w577 -> [w610 w632 w644 w668 _]
          tunnel: w574 -> [_ w623 w639 w663 _]
          tunnel: w573 -> [_ w624 w640 w664 _]
          tunnel: w570 -> [_ w629 w635 w654 _]
          tunnel: w569 -> [w606 w630 w642 w658 _]
          tunnel: w568 -> [_ w625 _ w657 _]
          tunnel: w567 -> [w600 w626 w637 w655 _]
          frame 0, Default {
            w611 = T1 {"Grid Type"=enum."Single Point", "Complex Convention"=enum."Re / Im", "Pattern Type"=enum."Rectangular", "Major Order Index"=0, "Grid Settings Value 1"=0.0+0.0i, "Grid Settings Value 2"=0.0+0.0i, "Pattern Settings Value 1"=0, "Pattern Settings Value 2"=0, "Values"=[0.0+0.0i]}  # Grid
            # "Single Point"
            n214 = case shown="0, Default" w607 {
              tunnel: w606 -> [w615 w616]
              tunnel: w600 -> [w614 w618]
              tunnel: [w613 w619] -> w605
              frame 0, Default {
                n215 = Re/Im To Complex(1:w614, 2:w615) -> (0:w613:cdb)
              }
              frame 1 {
                n216 = expression code="(x/180.0)*pi" ("degrees to radians")(w618) -> (w617:dbl)
                n217 = Polar To Complex(1:w617, 2:w616) -> (0:w619:cdb)
              }
            }
            n218 = Bundle By Name(cluster=w611, "Pattern Settings Value 2"=u32 0 ("patternSettingsValue 2"), "Pattern Settings Value 1"=u32 0 ("patternSettingsValue 1"), "Grid Settings Value 2"=cdb 0.0+0.0i ("gridSettingsValue 2"), "Grid Settings Value 1"=w605, "Major Order Index"=w610, "Pattern Type"=enum16{"Rectangular", "Circular", "Undefined"}."Rectangular" ("PatternType"), "Complex Convention"=w607, "Grid Type"=w608) -> (w601:T1)
          }
          frame 1 {
            w620 = T1 {"Grid Type"=enum."Single Point", "Complex Convention"=enum."Re / Im", "Pattern Type"=enum."Rectangular", "Major Order Index"=0, "Grid Settings Value 1"=0.0+0.0i, "Grid Settings Value 2"=0.0+0.0i, "Pattern Settings Value 1"=0, "Pattern Settings Value 2"=0, "Values"=[0.0+0.0i]}  # Grid
            # "Rectangle"
            n219 = Re/Im To Complex(1:w629, 2:w630) -> (0:w628:cdb)
            n220 = Re/Im To Complex(1:w625, 2:w626) -> (0:w627:cdb)
            n221 = Bundle By Name(cluster=w620, "Pattern Settings Value 2"=w623, "Pattern Settings Value 1"=w624, "Grid Settings Value 2"=w627, "Grid Settings Value 1"=w628, "Major Order Index"=w632, "Pattern Type"=w621, "Complex Convention"=enum16{"Re / Im", "Amp / Pha"}."Re / Im" ("ComplexConvention"), "Grid Type"=w631) -> (w633:T1)
          }
          frame 2 {
            w638 = T1 {"Grid Type"=enum."Single Point", "Complex Convention"=enum."Re / Im", "Pattern Type"=enum."Rectangular", "Major Order Index"=0, "Grid Settings Value 1"=0.0+0.0i, "Grid Settings Value 2"=0.0+0.0i, "Pattern Settings Value 1"=0, "Pattern Settings Value 2"=0, "Values"=[0.0+0.0i]}  # Grid
            # "Circle"
            n222 = case shown="0, Default" w641 {
              tunnel: w642 -> [w649 w650]
              tunnel: w637 -> [w648 w652]
              tunnel: [w647 w653] -> w636
              frame 0, Default {
                n223 = Re/Im To Complex(1:w648, 2:w649) -> (0:w647:cdb)
              }
              frame 1 {
                n224 = expression code="(x/180.0)*pi" ("degrees to radians")(w652) -> (w651:dbl)
                n225 = Polar To Complex(1:w651, 2:w650) -> (0:w653:cdb)
              }
            }
            n226 = Bundle By Name(cluster=w638, "Pattern Settings Value 2"=w639, "Pattern Settings Value 1"=w640, "Grid Settings Value 1"=w636, "Grid Settings Value 2"=w635, "Major Order Index"=w644, "Pattern Type"=w641, "Complex Convention"=w641, "Grid Type"=w643) -> (w645:T1)
          }
          frame 3 {
            w656 = T1 {"Grid Type"=enum."Single Point", "Complex Convention"=enum."Re / Im", "Pattern Type"=enum."Rectangular", "Major Order Index"=0, "Grid Settings Value 1"=0.0+0.0i, "Grid Settings Value 2"=0.0+0.0i, "Pattern Settings Value 1"=0, "Pattern Settings Value 2"=0, "Values"=[0.0+0.0i]}  # Grid
            # "Pie"
            n227 = expression code="(x/180.0)*pi" ("degrees to radians")(w657) -> (w660:dbl)
            n228 = expression code="(x/180.0)*pi" ("degrees to radians")(w654) -> (w659:dbl)
            n229 = Polar To Complex(1:w659, 2:w658) -> (0:w666:cdb)
            n230 = Polar To Complex(1:w660, 2:w655) -> (0:w665:cdb)
            n231 = Bundle By Name(cluster=w656, "Pattern Settings Value 2"=w663, "Pattern Settings Value 1"=w664, "Grid Settings Value 2"=w665, "Grid Settings Value 1"=w666, "Major Order Index"=w668, "Pattern Type"=w661, "Complex Convention"=enum16{"Re / Im", "Amp / Pha"}."Re / Im" ("ComplexConvention"), "Grid Type"=w667) -> (w669:T1)
          }
          frame 4 {
            w671 = T1 {"Grid Type"=enum."Single Point", "Complex Convention"=enum."Re / Im", "Pattern Type"=enum."Rectangular", "Major Order Index"=0, "Grid Settings Value 1"=0.0+0.0i, "Grid Settings Value 2"=0.0+0.0i, "Pattern Settings Value 1"=0, "Pattern Settings Value 2"=0, "Values"=[0.0+0.0i]}  # Grid
            n232 = property on="Custom Grid" class="Tbl (strict)"(error in=w677) -> (error out=w676:errorcluster, "Value"=w678:string[][])  [unwired: 1 in, 1 out]
            n233 = for {
              tunnel: w678 -> [w684] mode=indexing
              tunnel: w673 -> [w680]
              tunnel: [w679] -> w672 mode=indexing
              n234 = Index Array(array=w684, index=0 ("disabled index (col)")) -> (element=w689:string)
              n235 = Index Array(array=w684, index=1 ("disabled index (col)")) -> (element=w685:string)
              n236 = Scan From String(format string="%.;%f", input string=w689) -> (output 1=w681:dbl)  [unwired: 3 in, 3 out]
              n237 = Scan From String(format string="%.;%f", input string=w685) -> (output 1=w682:dbl)  [unwired: 3 in, 3 out]
              n238 = case shown="1" w680 {
                tunnel: w682 -> [w691 w694]
                tunnel: w681 -> [w692 w696]
                tunnel: [w690 w695] -> w679
                frame 0, Default {
                  n239 = Re/Im To Complex(1:w691, 2:w692) -> (0:w690:cdb)
                }
                frame 1 {
                  n240 = expression code="(x/180.0)*pi" ("degrees to radians")(w694) -> (w693:dbl)
                  n241 = Polar To Complex(1:w693, 2:w696) -> (0:w695:cdb)
                }
              }
            }
            n242 = Bundle By Name(cluster=w671, "Values"=w672, "Complex Convention"=w673, "Grid Type"=w675) -> (w674:T1)
          }
        }
        n243 = call "Generate Grid Values.vi"("Grid in"=w563) -> ("Grid out"=w562:T1)
        n244 = Unbundle By Name(w562) -> ("Values"=w566:cdb[])
        n245 = for {
          tunnel: w566 -> [w590] mode=indexing
          tunnel: [w596] -> w565 mode=indexing
          n246 = Add(x=cdb 1.0+0.0i, y=w590) -> (x+y=w594:cdb)
          n247 = Subtract(x=cdb 1.0+0.0i, y=w590) -> (x-y=w593:cdb)
          n248 = Divide(x=w594, y=w593) -> (x/y=w595:cdb)
          n249 = Complex To Re/Im(x + iy=w595) -> (x=w598:dbl, y=w597:dbl)
          n250 = Bundle(cluster=cluster{"r":dbl, "x":dbl} {"r"=0.2, "x"=0.3} ("Smith Pt"), "r"=w598, "x"=w597) -> (w596:cluster{"r":dbl, "x":dbl})
        }
        n251 = property on="Smith Chart" class="Pict"() -> ("Draw Area Size"=w587:T14)  [unwired: 2 in, 2 out]
        n252 = call <vilib>:"Smith Plot.vi"("smith plot"=w565, "dimensions (w,h)"=w587, "dimensions incl scales? (T)"=FALSE, "smith plot section"=T10 {"x minimum"=-1.1, "x maximum"=1.1, "y minimum"=-1.1, "y maximum"=1.1}, "smith plot cosmetics"=T12 {"Plot Style"=0, "Line Color"=0, "Point Color"=0}, "smith grid cosmetics"=T13 {"R color"=8355711, "R grids"=TRUE, "X color"=9868950, "X grids"=TRUE, "Labels"=FALSE}) -> ("new picture"=→"Smith Chart":picture)  [unwired: 9 in]
      }
    }
  }
  "Cancelled?" <- w10
  "Values" <- w6
  "Grid Settings Out" <- w5
  n253 = Merge Errors(w14, w13) -> (w12:errorcluster)
  n254 = Release Queue(queue=w11, error in (no error)=w12) -> (error out=→"error out":errorcluster)  [unwired: 1 in, 2 out]
